vi "Set Vertical Step Size.vi"(8 "error in":errorcluster, 10 "vertical step size":i16, 11 "eye scan in":refnum<class "niHighSpeedSerial Rectangular Eye Scan v1 Host.lvclass">) -> (0 "error out":errorcluster, 3 "eye scan out":refnum<class "niHighSpeedSerial Rectangular Eye Scan v1 Host.lvclass">)   [LabVIEW 2014, in "niHighSpeedSerial Rectangular Eye Scan v1 Host.lvclass"]
doc: "Sets the vertical step size. Valid values are between 1 and 127, inclusive.\n\n<B>Input Parameters</B>\n\n<B>eye scan in</B> Takes in a reference to your session from the previous VI.\n\n<B>vertical step size</B> is the number of offsets to skip between each point on the vertical axis.\n\n<B>error in</B> describes error conditions that occur before this node runs. This input provides standard 'error in' functionality.\n\n<B>Output Parameters</B>\n\n<B>eye scan out</B> passes a reference to your session to the next VI.\n\n<B>error out</B> contains error information. This output provides standard 'error out' functionality."
uses:
  <instrlib>/niHighSpeedSerial/Eye Scan/v1/Host/Impl/Rectangular Eye Scan/niHighSpeedSerial Rectangular Eye Scan v1 Host.lvclass
  <instrlib>/niHighSpeedSerial/Eye Scan/v1/Host/Impl/Rectangular Eye Scan/niHighSpeedSerial Rectangular Eye Scan v1 Host.lvclass/niHighSpeedSerial Rectangular Eye Scan v1 Host.ctl
  <vilib>/Utility/error.llb/Error Cluster From Error Code.vi
  <vilib>/ErrorRing/Error Ring.xnode
  <instrlib>/niHighSpeedSerial/Eye Scan/v1/Host/Eye Scan/niHighSpeedSerial Eye Scan v1 Host.lvclass
  <instrlib>/niHighSpeedSerial/Eye Scan/v1/Host/Common/niHighSpeedSerial Eye Scan Common v1 Host.lvlib
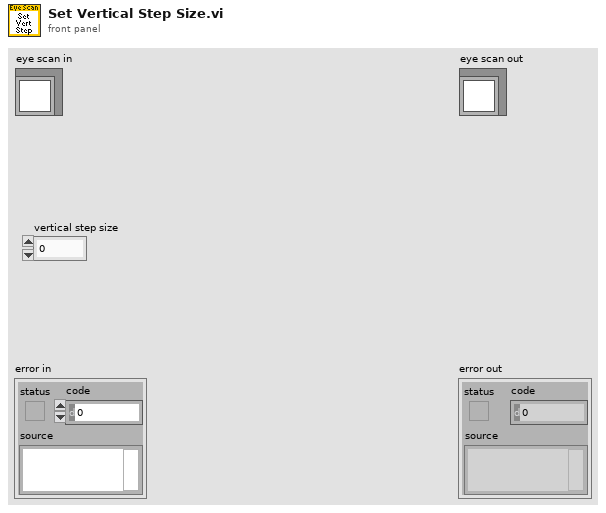
[diagram p1: front panel]
types:
  T1 = typedef "Rectangular Eye Scan v1 Host.lvclass/Private Data.ctl" = cluster{"horizontal step size":i16, "vertical step size":i16, "rectangular eye scan point iterator":refnum<class "niHighSpeedSerial Rectangular Eye Scan Point Iterator v1 Host.lvclass">}
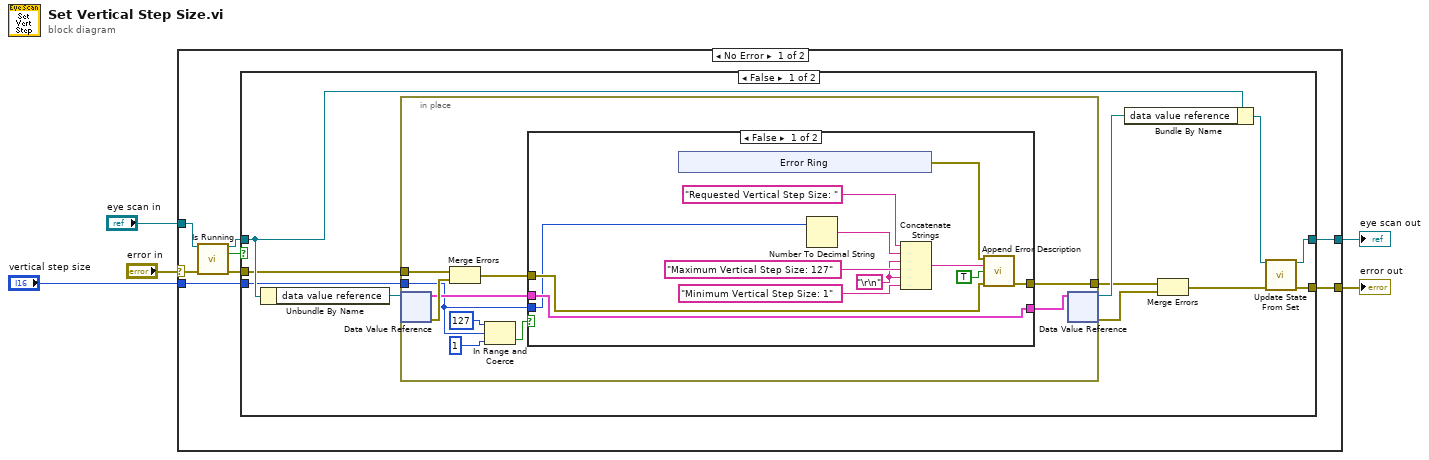
[diagram p0: block diagram]
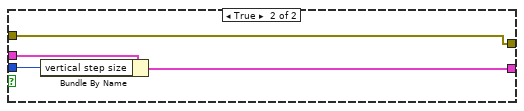
[diagram p2: hidden frame]
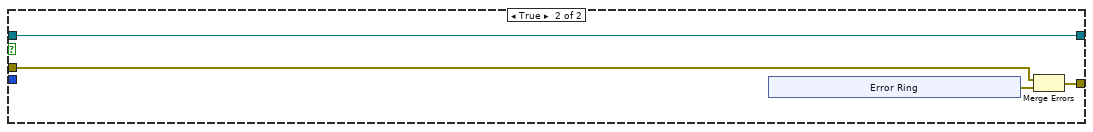
[diagram p3: hidden frame]
diagram:
  n1 = case shown="No Error" "error in" {
    selector: "error in" -> [w9 w64]
    tunnel: [w11 w64] -> w4
    tunnel: [w13 w63] -> w2
    tunnel: "eye scan in" -> [w7 w63]
    tunnel: "vertical step size" -> [w12 _]
    frame No Error {
      n2 = call <instrlib>:"Is Running.vi"("eye scan in"=w7, "error in"=w9) -> ("eye scan out"=w6:refnum<class "niHighSpeedSerial Rectangular Eye Scan v1 Host.lvclass">, "is running?"=w10:bool, "error out"=w8:errorcluster)  [unwired: 11 in]
      n3 = case shown="False" w10 {
        tunnel: [w14 w55] -> w13
        tunnel: w6 -> [w22 w55]
        tunnel: w12 -> [w21 _]
        tunnel: w8 -> [w20 w58]
        tunnel: [w16 w56] -> w11
        frame False {
          n4 = Unbundle By Name(w22) -> ("data value reference"=w24:refnum<data-value>)
          n5 = in-place {
            in-place-border: w21 -> [w25]
            in-place-border: w20 -> [w34]
            in-place-border: [w31] -> w18
            n6 = in-place-dvr #1(w24) -> (w27:T1, w33:errorcluster)
            n7 = Merge Errors(w34, w33) -> (w32:errorcluster)
            n8 = In Range and Coerce(upper limit=i16 127 ("x"), x=w25, lower limit=i16 1) -> (In Range?=w28:bool)  [unwired: 1 out]
            n9 = case shown="False" w28 {
              tunnel: [w35 w51] -> w31
              tunnel: w32 -> [w39 w51]
              tunnel: w27 -> [w37 w54]
              tunnel: [w37 w53] -> w26
              tunnel: w25 -> [w36 w52]
              frame False {
                w41 = "\r\n"
                n10 = xnode "Error Ring"() -> ("error out"=w46:errorcluster)
                n11 = Number To Decimal String(number=w36) -> (decimal integer string=w44:string)  [unwired: 1 in]
                n12 = Concatenate Strings("Requested Vertical Step Size: " ("append string (\"\")"), w44, w41, "Maximum Vertical Step Size: 127" ("string"), w41, "Minimum Vertical Step Size: 1" ("string")) -> (w43:string)
                n13 = call <instrlib>:"Append Error Description.vi"("error to append"=w46, "append string (\"\")"=w43, "generate error?"=TRUE, "error in"=w39) -> ("error out"=w35:errorcluster)  [unwired: 11 in]
              }
              frame True {
                n14 = Bundle By Name(cluster=w54, "vertical step size"=w52) -> (w53:T1)
              }
            }
            n15 = in-place-dvr #1(w26) -> (w23:refnum<data-value>, w19:errorcluster)
          }
          n16 = Bundle By Name(cluster=w22, "data value reference"=w23) -> (w15:refnum<class "niHighSpeedSerial Rectangular Eye Scan v1 Host.lvclass">)
          n17 = Merge Errors(w18, w19) -> (w17:errorcluster)
          n18 = call <instrlib>:"Update State From Set.vi"("eye scan in"=w15, "error in"=w17) -> ("eye scan out"=w14:refnum<class "niHighSpeedSerial Rectangular Eye Scan v1 Host.lvclass">, "error out"=w16:errorcluster)  [unwired: 12 in]
        }
        frame True {
          n19 = xnode "Error Ring"() -> ("error out"=w57:errorcluster)
          n20 = Merge Errors(w58, w57) -> (w56:errorcluster)
        }
      }
    }
    frame Error {
    }
  }
  "error out" <- w4
  "eye scan out" <- w2
